vi "Configure Data Interleave.vi"(6 "Data Interleave (1)":i32=1, 7 "Channel (1: Channel 1)":i32(ring)=1 items=["All"=0, "Channel 1"=1, "Channel 1.1"=11, "Channel 1.2"=12, "Channel 1.3"=13, "Channel 1.4"=14, "Channel 2"=2, "Channel 2.1"=21, "Channel 2.2"=22, "Channel 2.3"=23, "Channel 2.4"=24, "Channel 3"=3, "Channel 3.1"=31, "Channel 3.2"=32, "Channel 3.3"=33, "Channel 3.4"=34, "Channel 4"=4, "Channel 4.1"=41, "Channel 4.2"=42, "Channel 4.3"=43, "Channel 4.4"=44], 8 "error in (no error)":errorcluster, 9 "Number of Averages (1)":i32=1, 10 "Sensor Number (1)":i32=1, 11 "VISA resource name":refnum<visa-resource-name>) -> (0 "error out":errorcluster, 3 "VISA resource name out":refnum<visa-resource-name>)   [LabVIEW 2024, in "Micron Optics sm130.lvlib"]
doc: "Configures data interleave and number of averages to specified channel and sensor. \n\n<b>Note:</b>\nBy using data interleave, the instrument continues to acquire data at its full rate while only reporting data at a reduced rate as determined by Data Interleave Parameter. Asthe module continues to acquire at max rate, data is available between periods of reporting to facilitate averaging. Averaging reduces the noise of the measurement."
uses:
  Micron Optics sm130.lvlib
panel:
  out "Confirmation Response 2":string
  out "Confirmation Response":string
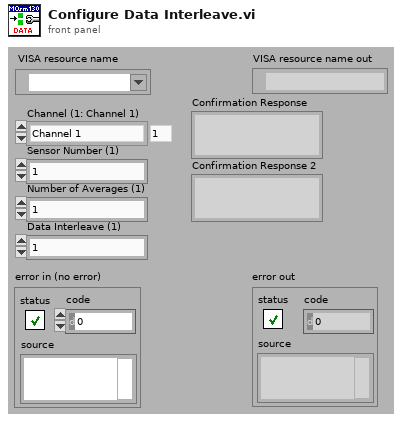
[diagram p1: front panel]
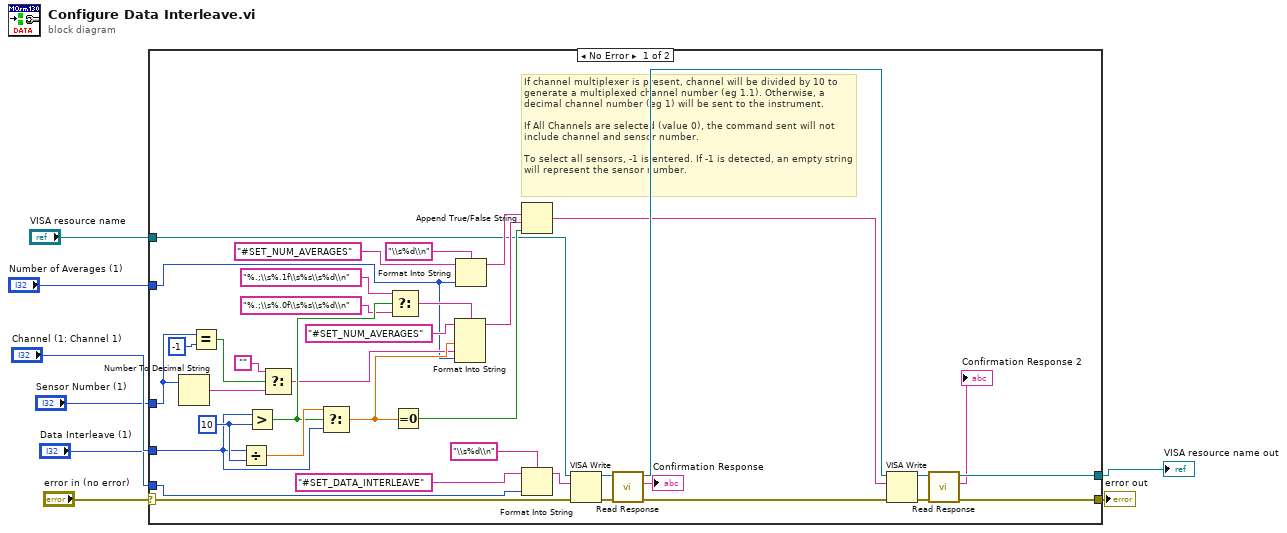
[diagram p0: block diagram]
diagram:
  n1 = case shown="No Error" "error in (no error)" {
    selector: "error in (no error)" -> [w11 w48]
    tunnel: "Channel (1: Channel 1)" -> [w37 _]
    tunnel: "Sensor Number (1)" -> [w32 _]
    tunnel: "Number of Averages (1)" -> [w29 _]
    tunnel: "Data Interleave (1)" -> [w20 _]
    tunnel: "VISA resource name" -> [w14 w47]
    tunnel: [w13 w47] -> w3
    tunnel: [w12 w48] -> w2
    frame No Error {
      w45 = 10 ("y")
      # "If channel multiplexer is present, channel will be divided by 10 to generate a multiplexed channel number (eg 1.1). Otherwise, a decimal channel number (eg 1) will be sent to the instrument.\n\nIf All Channels are selected (value 0), the command sent will not include channel and sensor number. \n \nTo select all sensors, -1 is entered. If -1 is detected, an empty string will represent the sensor number."
      n2 = Number To Decimal String(number=w32) -> (decimal integer string=w33:string)  [unwired: 1 in]
      n3 = Equal?(x=w32, y=-1) -> (x = y?=w35:bool)
      n4 = Divide(x=w37, y=w45) -> (x/y=w46:dbl)
      n5 = Greater?(x=w37, y=w45) -> (0:w44:bool)
      n6 = Select(t="", s=w35, f=w33) -> (s? t:f=w31:string)
      n7 = Select(t=w46, s=w44, f=w37) -> (s? t:f=w40:dbl)
      n8 = Select(t="%.;\\s%.1f\\s%s\\s%d\\n" ("format string"), s=w44, f="%.;\\s%.0f\\s%s\\s%d\\n" ("format string")) -> (s? t:f=w41:string)
      n9 = Equal To 0?(x=w40) -> (x = 0?=w38:bool)
      n10 = Format Into String(format string=w41, initial string="#SET_NUM_AVERAGES", w40, w31, w29) -> (resulting string=w39:string)  [unwired: 1 in, 1 out]
      n11 = Format Into String(format string="\\s%d\\n", initial string="#SET_NUM_AVERAGES", w29) -> (resulting string=w27:string)  [unwired: 1 in, 1 out]
      n12 = Append True/False String(1:w38, 2:w39, 3:w27) -> (0:w15:string)  [unwired: 1 in]
      n13 = Format Into String(format string="\\s%d\\n", initial string="#SET_DATA_INTERLEAVE", w20) -> (resulting string=w21:string)  [unwired: 1 in, 1 out]
      n14 = VISA Write(VISA resource name=w14, write buffer=w21, error in (no error)=w11) -> (VISA resource name out=w23:refnum<visa-resource-name>, error out=w22:errorcluster)  [unwired: 1 out]
      n15 = call "Read Response.vi"("error in (no error)"=w22, "VISA resource name"=w23) -> ("error out"=w17:errorcluster, "Confirmation Response"=→"Confirmation Response":string, "VISA resource name out"=w16:refnum<visa-resource-name>)  [unwired: 7 in]
      n16 = VISA Write(VISA resource name=w16, write buffer=w15, error in (no error)=w17) -> (VISA resource name out=w18:refnum<visa-resource-name>, error out=w19:errorcluster)  [unwired: 1 out]
      n17 = call "Read Response.vi"("error in (no error)"=w19, "VISA resource name"=w18) -> ("error out"=w12:errorcluster, "Confirmation Response"=→"Confirmation Response 2":string, "VISA resource name out"=w13:refnum<visa-resource-name>)  [unwired: 7 in]
    }
    frame Error {
    }
  }
  "VISA resource name out" <- w3
  "error out" <- w2
